vi "generateSimulatedData.vi"(8 "error in (no error)":errorcluster, 11 "DistanceGaugeSim in":refnum<class "DistanceGaugeSim.lvclass">) -> (0 "error out":errorcluster, 2 "stringRead":string, 3 "DistanceGaugeSim out":refnum<class "DistanceGaugeSim.lvclass">)   [LabVIEW 2013, in "DistanceGaugeSim.lvclass"]
uses:
  DistanceGaugeSim.lvclass
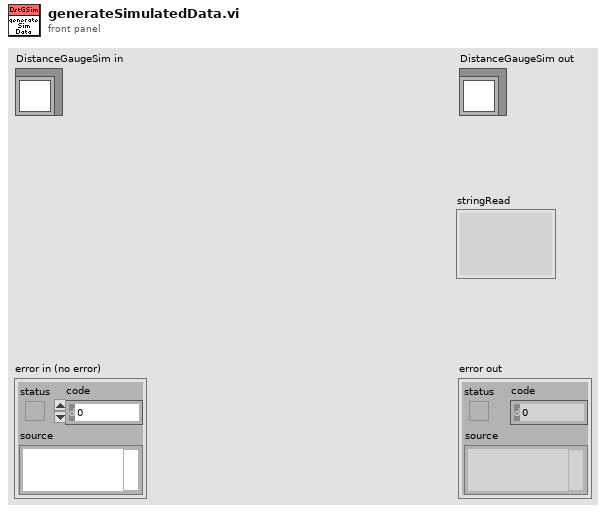
[diagram p1: front panel]
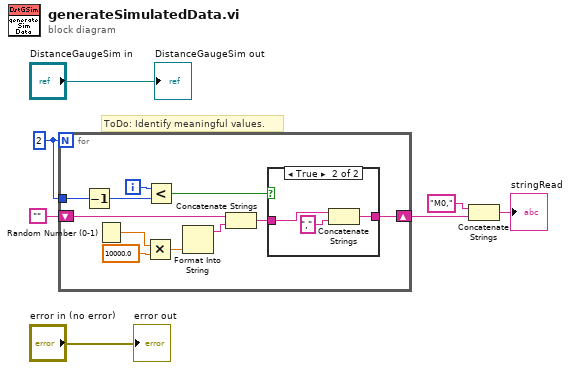
[diagram p0: block diagram]
diagram:
  w4 = 2
  # "ToDo: Identify meaningful values."
  n1 = for {
    N: w4 -> [_]
    shift-right: [w12] -> w3
    shift-left: "" -> [w15]
    tunnel: w4 -> [w10]
    i -> [w11]
    n2 = Decrement(x=w10) -> (x-1=w9:i32)
    n3 = Random Number (0-1)() -> (number: 0 to 1=w18:dbl)
    n4 = Multiply(x=w18, y=10000.0) -> (x*y=w16:dbl)
    n5 = Less?(x=w11, y=w9) -> (x < y?=w8:bool)
    n6 = Format Into String(w16) -> (resulting string=w14:string)  [unwired: 3 in, 1 out]
    n7 = Concatenate Strings(w15, w14) -> (w13:string)
    n8 = case shown="True" w8 {
      tunnel: w13 -> [w19 w22]
      tunnel: [w19 w20] -> w12
      frame False {
      }
      frame True {
        n9 = Concatenate Strings(w22, "," ("string")) -> (w20:string)
      }
    }
  }
  n10 = Concatenate Strings("M0," ("string"), w3) -> (→"stringRead":string)
  "error out" <- "error in (no error)"
  "DistanceGaugeSim out" <- "DistanceGaugeSim in"
